vi "Collect Data.vi"(8 "error in (no error)":errorcluster, 10 "AbstractData in":refnum<class "AbstractData.lvclass">, 11 "AbstractCollector2D in":refnum<class "AbstractCollector2D.lvclass">) -> (0 "error out":errorcluster, 2 "finished?":bool=TRUE, 3 "AbstractCollector2D out":refnum<class "AbstractCollector2D.lvclass">)   [LabVIEW 2014, in "AbstractCollector2D.lvclass"]
uses:
  AbstractCollector2D.lvclass
  Model/Data/AbstractData/AbstractData.lvclass
  Model/Data/Data2D/Data2D.lvclass
  Data2D Cluster.ctl
  AbstractCollector/AbstractCollector.lvclass
  Interfaces/Observable Actor/Observable Actor.lvclass
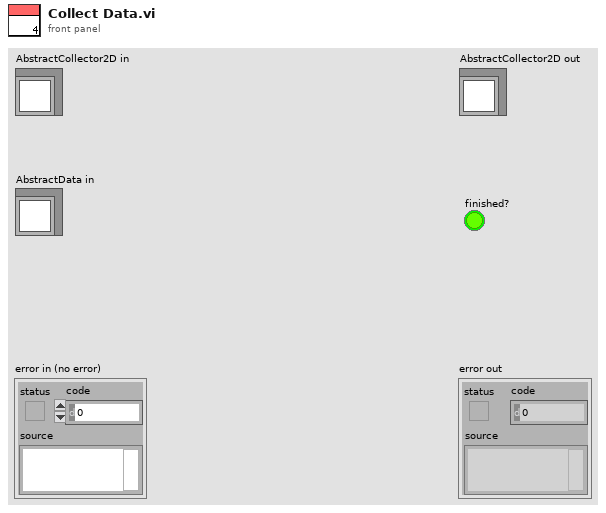
[diagram p1: front panel]
types:
  T1 = typedef "AbstractCollector2D.lvclass/Data2D Cluster.ctl" = cluster{"in":refnum<class "Data2D.lvclass">, "intermediate":refnum<class "Data2D.lvclass">}
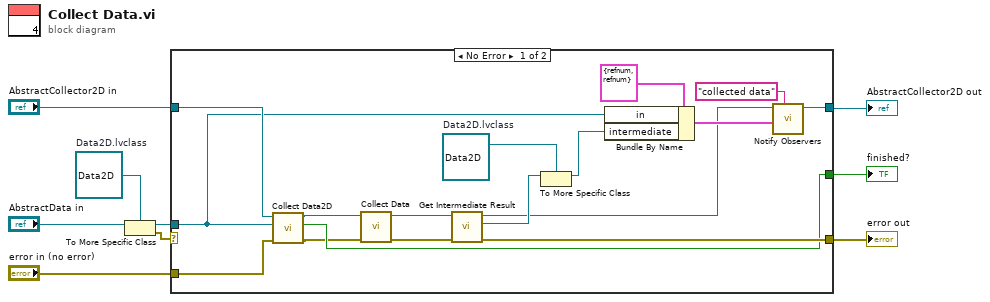
[diagram p0: block diagram]
diagram:
  w1 = refnum<class "Data2D.lvclass"> refnum  # Data2D.lvclass
  n1 = To More Specific Class(target class=w1, reference="AbstractData in") -> (specific class reference=w8:refnum<class "Data2D.lvclass">, error out=w9:errorcluster)  [unwired: 1 in]
  n2 = case shown="No Error" w9 {
    tunnel: w8 -> [w11 _]
    tunnel: "error in (no error)" -> [w13 w28]
    tunnel: [w22 w28] -> w3
    tunnel: "AbstractCollector2D in" -> [w12 w27]
    tunnel: [w24 w27] -> w5
    tunnel: [w15 _] -> w6
    frame No Error {
      w17 = refnum<class "Data2D.lvclass"> refnum  # Data2D.lvclass
      n3 = call-dynamic "Collect Data2D.vi"("error in (no error)"=w13, "Data2D in"=w11, "AbstractCollector2D in"=w12) -> ("error out"=w14:errorcluster, "finished?"=w15:bool, "AbstractCollector2D out"=w16:refnum<class "AbstractCollector2D.lvclass">)  [unwired: 6 in]
      n4 = call-parent "Collect Data.vi"("error in (no error)"=w14, "AbstractCollector in"=w16) -> ("error out"=w18:errorcluster, "AbstractCollector out"=w19:refnum<class "AbstractCollector2D.lvclass">)  [unwired: 7 in, 1 out]
      n5 = call-dynamic "Get Intermediate Result.vi"("error in (no error)"=w18, "AbstractCollector in"=w19) -> ("error out"=w22:errorcluster, "AbstractData.lvclass"=w26:refnum<class "AbstractData.lvclass">, "AbstractCollector out"=w21:refnum<class "AbstractCollector2D.lvclass">)  [unwired: 7 in]
      n6 = To More Specific Class(target class=w17, reference=w26) -> (specific class reference=w25:refnum<class "Data2D.lvclass">)  [unwired: 1 in, 1 out]
      n7 = Bundle By Name(cluster=T1 {"in"=refnum, "intermediate"=refnum}, "in"=w11, "intermediate"=w25) -> (w23:T1)
      n8 = call "Notify Observers.vi"("name"="collected data", "value"=w23, "Observable Actor in"=w21) -> ("Observable Actor out"=w24:refnum<class "AbstractCollector2D.lvclass">)  [unwired: 7 in, 1 out]
    }
    frame Error {
    }
  }
  "error out" <- w3
  "AbstractCollector2D out" <- w5
  "finished?" <- w6
